vi "Pneumatics Command Set Periodic.vi"(10 "Solenoid Command":T2, 11 "Cluster":T1) -> (3 "Cluster Out":T1)   [LabVIEW 2015]
uses:
  Pneumatics Notifier.ctl
  Pneumatics Command.ctl
  Pneumatics Status.ctl
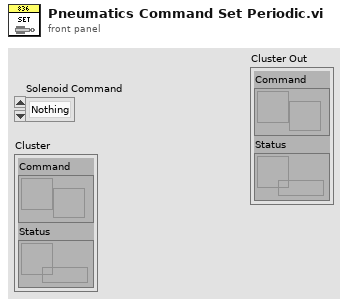
[diagram p1: front panel]
types:
  T1 = typedef "Pneumatics Notifier.ctl" = cluster{"Command":refnum<notifier>, "Status":refnum<queue>}
  T2 = typedef "Pneumatics Command.ctl" = enum16{"Nothing", "Forward", "Reverse", "Toggle"}
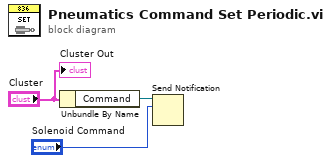
[diagram p0: block diagram]
diagram:
  n1 = Unbundle By Name("Cluster") -> ("Command"=w2:refnum<notifier>)
  n2 = Send Notification(notification="Solenoid Command", notifier=w2) -> ()  [unwired: 1 in, 2 out]
  "Cluster Out" <- "Cluster"
